vi "Process_Errors.vi"(6 "Queues":T1, 8 "Status/Errors in":refnum<vi>) -> (0 "Status/Errors out":refnum<vi>)   [LabVIEW 2010]
uses:
  Controls/Queues.ctl
  Controls/One_Second.ctl
  Controls/GPS_Timestamp.ctl
  Controls/Master.ctl
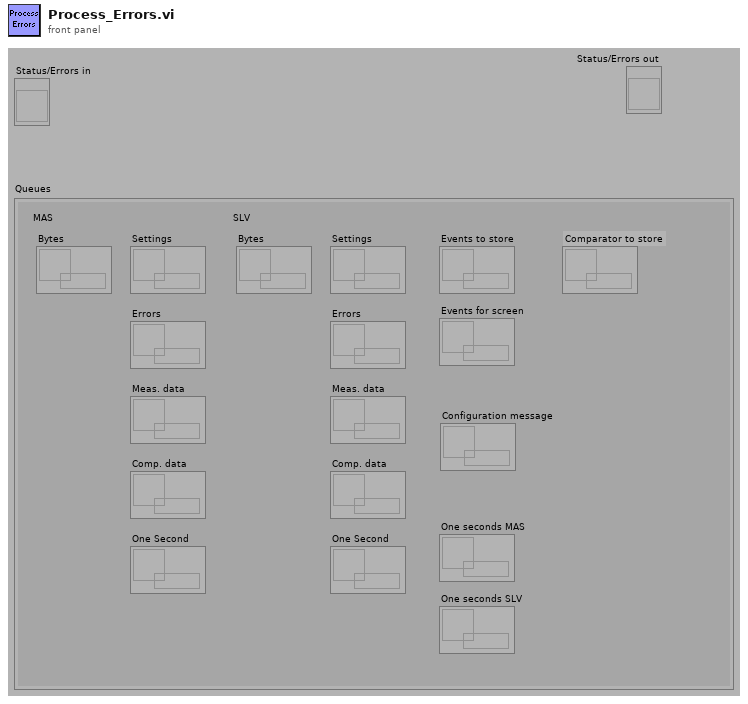
[diagram p1: front panel]
types:
  T1 = typedef "Queues.ctl" = cluster{"MAS":cluster{"Bytes":refnum<queue>, "Settings":refnum<queue>, "Errors":refnum<queue>, "Meas. data":refnum<queue>, "One Second":refnum<queue>, "Comp. data":refnum<queue>}, "SLV":cluster{"Bytes":refnum<queue>, "Settings":refnum<queue>, "Errors":refnum<queue>, "Meas. data":refnum<queue>, "One Second":refnum<queue>, "Comp. data":refnum<queue>}, "Events to store":refnum<queue>, "Events for screen":refnum<queue>, "One seconds MAS":refnum<queue>, "One seconds SLV":refnum<queue>, "Configuration message":refnum<queue>, "Comparator to store":refnum<queue>}
  T2 = typedef "Master.ctl" = enum16{"Master", "Slave", "General"}
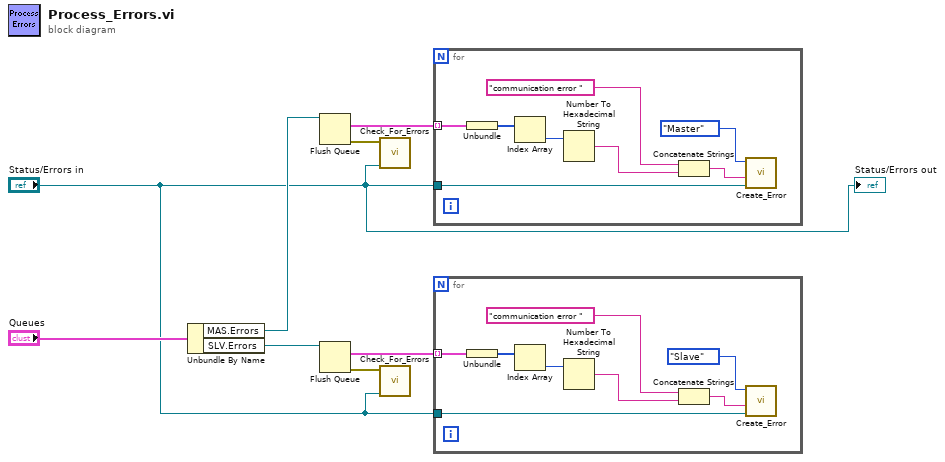
[diagram p0: block diagram]
diagram:
  n1 = Unbundle By Name("Queues") -> ("MAS.Errors"=w7:refnum<queue>, "SLV.Errors"=w2:refnum<queue>)
  n2 = Flush Queue(queue=w7) -> (remaining elements=w6:cluster{u8[]}[], error out=w5:errorcluster)  [unwired: 1 in, 1 out]
  n3 = Flush Queue(queue=w2) -> (remaining elements=w4:cluster{u8[]}[], error out=w3:errorcluster)  [unwired: 1 in, 1 out]
  n4 = call "Check_For_Errors.vi"("Status/Errors in"="Status/Errors in", "error in"=w5) -> ()  [unwired: 10 out]
  n5 = call "Check_For_Errors.vi"("Status/Errors in"="Status/Errors in", "error in"=w3) -> ()  [unwired: 10 out]
  n6 = for {
    tunnel: w6 -> [w16] mode=indexing
    tunnel: "Status/Errors in" -> [w13]
    n7 = Unbundle(w16) -> (w15:u8[])
    n8 = Index Array(array=w15) -> (element=w10:u8)  [unwired: 1 in]
    n9 = Number To Hexadecimal String(2:w10) -> (0:w9:string)  [unwired: 1 out]
    n10 = Concatenate Strings("communication error " ("HiSPARC error"), w9) -> (w12:string)
    n11 = call "Create_Error.vi"("Status/Errors in"=w13, "HiSPARC error"=w12, "Master?"=Master."Master") -> ()  [unwired: 3 in, 6 out]
  }
  n12 = for {
    tunnel: w4 -> [w24] mode=indexing
    tunnel: "Status/Errors in" -> [w21]
    n13 = Unbundle(w24) -> (w23:u8[])
    n14 = Index Array(array=w23) -> (element=w18:u8)  [unwired: 1 in]
    n15 = Number To Hexadecimal String(2:w18) -> (0:w17:string)  [unwired: 1 out]
    n16 = Concatenate Strings("communication error " ("HiSPARC error"), w17) -> (w20:string)
    n17 = call "Create_Error.vi"("Status/Errors in"=w21, "HiSPARC error"=w20, "Master?"=Master."Slave") -> ()  [unwired: 3 in, 6 out]
  }
  "Status/Errors out" <- "Status/Errors in"
